vi "Set Device Coupling.vi"(8 "Error In (none)":errorcluster, 9 "Bus Selector (both)":enum16{"primary", "secondary", "both"}(ring)=enum."both", 10 "Coupling Mode (isolated)":T1, 11 "Module Handle":u32) -> (0 "Error Out":errorcluster, 3 "Module Handle out":u32)   [LabVIEW 2020, in "AIM MIL-STD-1553 Hardware API.lvlib"]
doc: "<B>Input Parameters:</B>\n\nModule Handle - Reference to the device as obtained from a call to: 1553 General - Obtain a Device Reference.vi\n\nBIU Number (1) - BIU number (one-based) of the bus interface unit.\n\n<B> Output Parameters: </B>"
uses:
  AIM MIL-STD-1553 Hardware API.lvlib
  <instrlib>/_AIM MIL-STD-1553/AIM Controls/1553 Couplingmodes.ctl
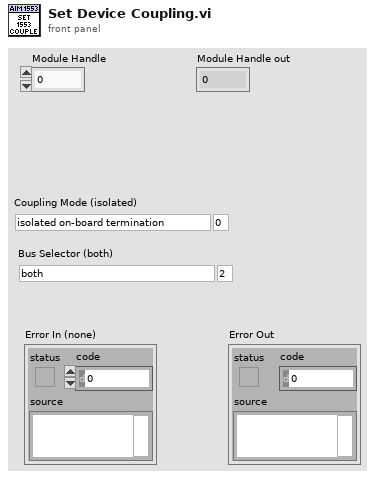
[diagram p1: front panel]
types:
  T1 = typedef "1553 Couplingmodes.ctl" = enum16{"isolated on-board termination", "transformer coupled", "direct coupled", "external with on-board termination", "on-board digital wrap-around"}
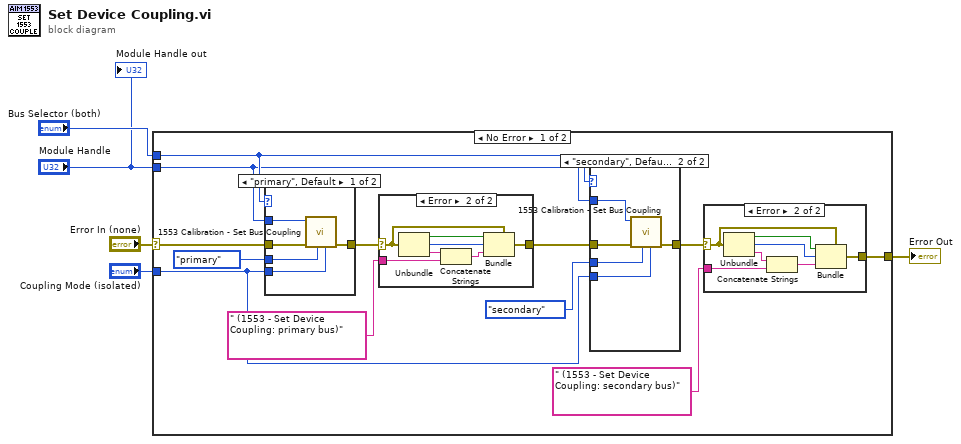
[diagram p0: block diagram]
diagram:
  n1 = case shown="No Error" "Error In (none)" {
    selector: "Error In (none)" -> [w17 w46]
    tunnel: [w14 w46] -> w4
    tunnel: "Module Handle" -> [w8 _]
    tunnel: "Coupling Mode (isolated)" -> [w12 _]
    tunnel: "Bus Selector (both)" -> [w9 _]
    frame No Error {
      n2 = case shown="\"primary\", Default" w9 {
        tunnel: w17 -> [w28 w29]
        tunnel: enum16{"primary", "secondary"}."primary" ("Bus (primary)") -> [w27 _]
        tunnel: w8 -> [w26 _]
        tunnel: w12 -> [w25 _]
        tunnel: [w24 w29] -> w15
        frame "primary", Default {
          n3 = call <instrlib>:"1553 Calibration - Set Bus Coupling.vi"("Coupling Mode (isolated)"=w25, "Bus (primary)"=w27, "Error In (none)"=w28, "Module Handle"=w26) -> ("Error Out"=w24:errorcluster)  [unwired: 7 in]
        }
        frame "secondary" {
        }
      }
      n4 = case shown="Error" w15 {
        selector: w15 -> [w38 w44]
        tunnel: [w38 w45] -> w11
        tunnel: " (1553 - Set Device Coupling: primary bus)" ("source") -> [_ w39]
        frame No Error {
        }
        frame Error {
          n5 = Unbundle(w44) -> ("status"=w43:bool, "code"=w42:i32, "source"=w41:string)
          n6 = Concatenate Strings(w41, w39) -> (w40:string)
          n7 = Bundle(cluster=w44, "status"=w43, "code"=w42, "source"=w40) -> (w45:errorcluster)
        }
      }
      n8 = case shown="\"secondary\", Default" w9 {
        tunnel: w11 -> [w18 w23]
        tunnel: enum16{"primary", "secondary"}."secondary" ("Bus (primary)") -> [_ w22]
        tunnel: w8 -> [_ w21]
        tunnel: w12 -> [_ w20]
        tunnel: [w18 w19] -> w10
        frame "primary" {
        }
        frame "secondary", Default {
          n9 = call <instrlib>:"1553 Calibration - Set Bus Coupling.vi"("Coupling Mode (isolated)"=w20, "Bus (primary)"=w22, "Error In (none)"=w23, "Module Handle"=w21) -> ("Error Out"=w19:errorcluster)  [unwired: 7 in]
        }
      }
      n10 = case shown="Error" w10 {
        selector: w10 -> [w30 w36]
        tunnel: [w30 w37] -> w14
        tunnel: " (1553 - Set Device Coupling: secondary bus)" ("source") -> [_ w31]
        frame No Error {
        }
        frame Error {
          n11 = Unbundle(w36) -> ("status"=w35:bool, "code"=w34:i32, "source"=w33:string)
          n12 = Concatenate Strings(w33, w31) -> (w32:string)
          n13 = Bundle(cluster=w36, "status"=w35, "code"=w34, "source"=w32) -> (w37:errorcluster)
        }
      }
    }
    frame Error {
    }
  }
  "Error Out" <- w4
  "Module Handle out" <- "Module Handle"
